vi "Read FIFO Pub.vi"(8 "error in":errorcluster, 11 "ChanMngOOB_Rx in":refnum<class "ChanMngOOB_Rx.lvclass">) -> (0 "error out":errorcluster, 2 "FIFO Pub":T1, 3 "ChanMngOOB_Rx out":refnum<class "ChanMngOOB_Rx.lvclass">)   [LabVIEW 2021, in "ChanMngOOB_Rx.lvclass"]
uses:
  ChanMngOOB_Rx.lvclass
  ChanMngOOB_Rx.lvclass/ChanMngOOB_Rx.ctl
  <vilib>/CIF Foundation/CIF Channels Core/ChannelCommon/typedef/New FIFO Instance Configuration.ctl
  <vilib>/CIF Foundation/CIF Channels Core/ChannelCommon/ChannelCommon.lvlib
  Typedef/FIFO Publisher.ctl
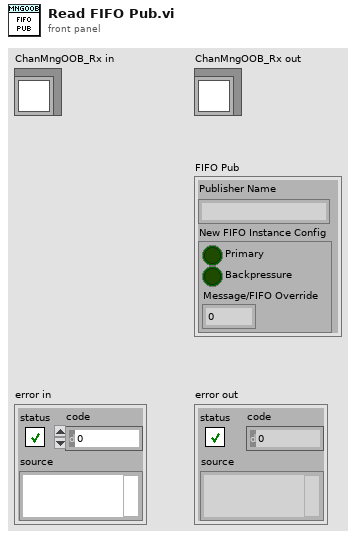
[diagram p1: front panel]
types:
  T1 = typedef "ChanMngOOB_Rx.lvclass/FIFO Publisher.ctl" = cluster{"Publisher Name":string, "New FIFO Instance Config":T2}
  T2 = typedef "ChannelCommon.lvlib/New FIFO Instance Configuration.ctl" = cluster{"Primary":bool, "Backpressure":bool, "Message/FIFO Override":u32}
  T3 = typedef "ChanMngOOB_Rx.lvclass/Template Payload.ctl" = cluster{"Connections":T4[], "Forces":T5[], "FIFO Pub":T1}
  T4 = typedef "ChanMngOOB_Rx.lvclass/Channel Connection Data.ctl" = cluster{"Publisher Name":string, "Subscriber Name":string, "Connection Data":u8[]}
  T5 = typedef "ChanMngOOB_Rx.lvclass/Channel Fault Data.ctl" = cluster{"Channel Name":string, "Force Data":u8[], "Force Active":bool}
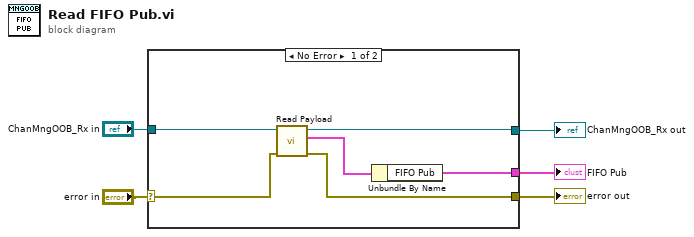
[diagram p0: block diagram]
diagram:
  n1 = case shown="No Error" "error in" {
    selector: "error in" -> [w11 w13]
    tunnel: [w9 w13] -> w5
    tunnel: [w6 w12] -> w4
    tunnel: "ChanMngOOB_Rx in" -> [w8 w12]
    tunnel: [w7 _] -> w1
    frame No Error {
      n2 = call "Read Payload.vi"("error in"=w11, "ChanMngOOB_Rx in"=w8) -> ("error out"=w9:errorcluster, "data"=w10:T3, "ChanMngOOB_Rx out"=w6:refnum<class "ChanMngOOB_Rx.lvclass">)  [unwired: 7 in]
      n3 = Unbundle By Name(w10) -> ("FIFO Pub"=w7:T1)
    }
    frame Error {
    }
  }
  "error out" <- w5
  "ChanMngOOB_Rx out" <- w4
  "FIFO Pub" <- w1
